vi "Configure AC Line Trigger Slope [AT] Core.vi"(8 "error in (no error)":errorcluster, 10 "ac line trigger slope (Positive)":i32(ring)=1 items=["Positive"=1, "Negative"=2, "Either"=3], 11 "CS++Scope":refnum<class "CS++Scope.lvclass">) -> (0 "error out":errorcluster, 3 "CS++Scope out":refnum<class "CS++Scope.lvclass">)   [LabVIEW 2015, in "CS++Scope.lvlib" / "CS++Scope.lvclass"]
doc: "This VI configures the slope of the AC Line trigger.\n\nNote (1) This VI affects instrument behavior only if the trigger type is IVISCOPE_VAL_AC_LINE_TRIGGER. Call the IviScope Configure Trigger VI to set the trigger type before calling this VI.\n(2) This VI is part of the IviScopeAcLineTrigger [AT] extension group."
uses:
  CS++Scope.lvclass
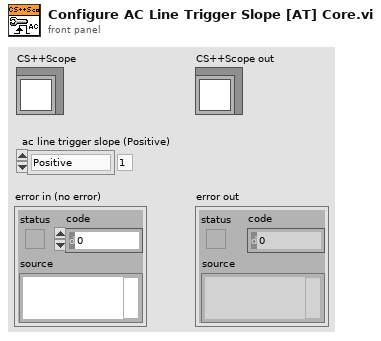
[diagram p1: front panel]
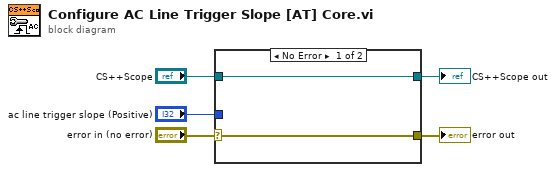
[diagram p0: block diagram]
diagram:
  n1 = case shown="No Error" "error in (no error)" {
    selector: "error in (no error)" -> [w6 w9]
    tunnel: [w6 w9] -> w4
    tunnel: [w7 w8] -> w2
    tunnel: "CS++Scope" -> [w7 w8]
    tunnel: "ac line trigger slope (Positive)" -> [_ _]
    frame No Error {
    }
    frame Error {
    }
  }
  "error out" <- w4
  "CS++Scope out" <- w2
